vi "write buffer Date.vi"(8 "error in (no error)":errorcluster caption="错误输入（无错误）", 10 "写入缓冲区":string, 11 "串口参数管理 输入":refnum<class "串口通讯.lvclass">) -> (0 "error out":errorcluster caption="错误输出", 3 "串口参数管理 输出":refnum<class "串口通讯.lvclass">)   [LabVIEW 2015, in "串口通讯.lvlib" / "串口通讯.lvclass"]
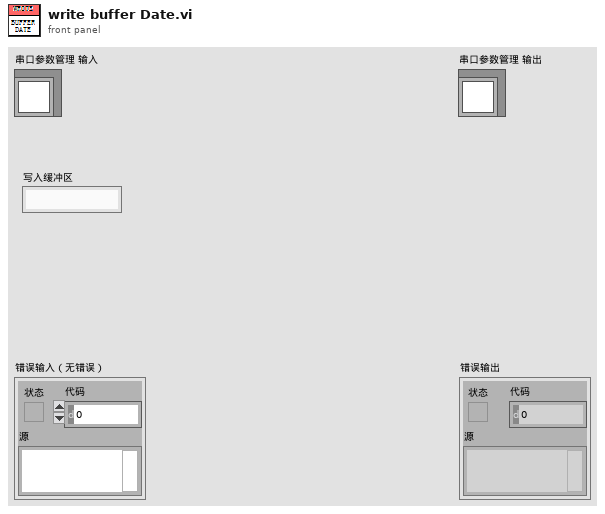
[diagram p1: front panel]
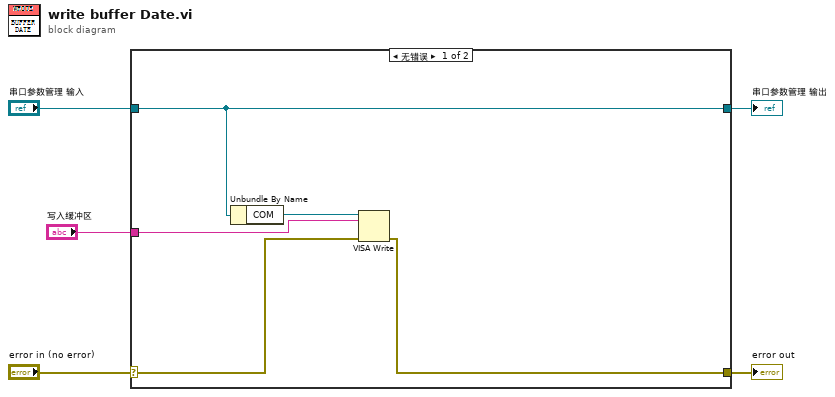
[diagram p0: block diagram]
diagram:
  n1 = case shown="无错误" "error in (no error)" {
    selector: "error in (no error)" -> [w8 w12]
    tunnel: [w7 w12] -> w4
    tunnel: [w10 w11] -> w2
    tunnel: "串口参数管理 输入" -> [w10 w11]
    tunnel: "写入缓冲区" -> [w6 _]
    frame No Error {
      n2 = Unbundle By Name(w10) -> ("COM"=w9:refnum<visa-resource-name>)
      n3 = VISA Write(VISA resource name=w9, write buffer=w6, error in (no error)=w8) -> (error out=w7:errorcluster)  [unwired: 2 out]
    }
    frame Error {
    }
  }
  "error out" <- w4
  "串口参数管理 输出" <- w2
